vi "set top index.vi"(8 "error in (no error)":errorcluster, 10 "Numeric":u32, 11 "Array in":refnum<vi>) -> (0 "error out":errorcluster, 3 "Array out":refnum<vi>)   [LabVIEW 2014, in "PID Module editor node.lvclass"]
uses:
  PID Module editor node.lvclass
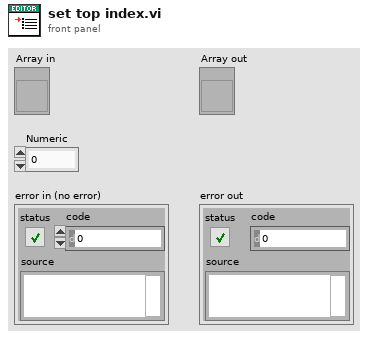
[diagram p1: front panel]
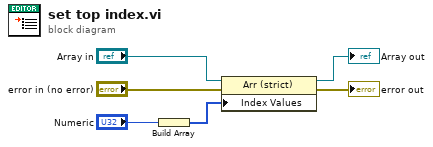
[diagram p0: block diagram]
diagram:
  n1 = Build Array("Numeric") -> (w5:u32[])
  n2 = property class="Arr (strict)"(reference="Array in", error in="error in (no error)", "Index Values"=w5) -> (reference out=→"Array out":refnum<vi>, error out=→"error out":errorcluster)
